vi "StopAllMotion.vi"(0 "System no.":i32, 2 "Has #24":bool=TRUE, 5 "error in (no error)":errorcluster) -> (19 "error out":errorcluster)   [LabVIEW 2020]
doc: "A Support VI to Stop all motion. It takes some controller and syntax specific behavior into account"
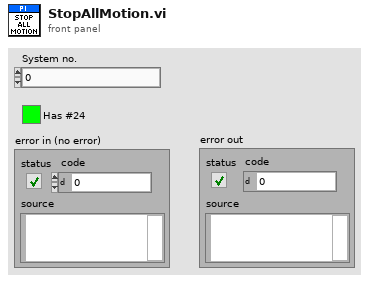
[diagram p1: front panel]
types:
  T1 = typedef "Syntax.ctl" = enum16{"GCS 1.0", "GCS 2.0", "GCS 3.0"}
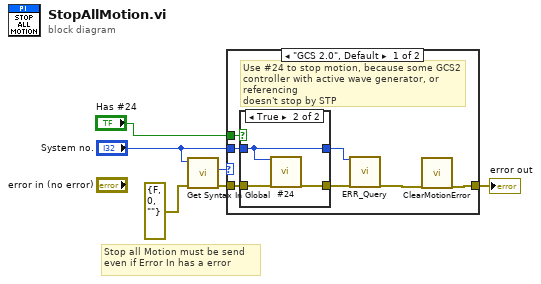
[diagram p0: block diagram]
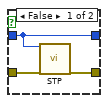
[diagram p2: hidden frame]
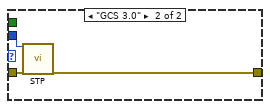
[diagram p3: hidden frame]
diagram:
  # "Stop all Motion must be send\neven if Error In has a error"
  n1 = call "Get Syntax In Global.vi"("error in"=errorcluster {"status"=FALSE, "code"=0, "source"=""}, "System no."="System no.") -> ("error out"=w5:errorcluster, "Syntax"=w4:T1)  [unwired: 8 in]
  n2 = case shown="\"GCS 2.0\", Default" w4 {
    tunnel: [w7 w20] -> w6
    tunnel: "System no." -> [w13 w21]
    tunnel: w5 -> [w12 w22]
    tunnel: "Has #24" -> [w10 _]
    frame "GCS 2.0", Default {
      # "Use #24 to stop motion, because some GCS2 controller with active wave generator, or referencing \ndoesn't stop by STP"
      n3 = case shown="True" w10 {
        tunnel: w13 -> [w14 w17]
        tunnel: w12 -> [w16 w19]
        tunnel: [w15 w18] -> w11
        tunnel: [w14 w17] -> w9
        frame False {
          n4 = call "STP.vi"("System no."=w14, "error in"=w16) -> ("error out"=w15:errorcluster)  [unwired: 17 in]
        }
        frame True {
          n5 = call "#24.vi"("System no."=w17, "error in"=w19) -> ("error out"=w18:errorcluster)  [unwired: 17 out]
        }
      }
      n6 = call "ERR_Query.vi"("System no."=w9, "error in"=w11) -> ("error out"=w8:errorcluster)  [unwired: 17 out]
      n7 = call "ClearMotionError.vi"("error in (no error)"=w8) -> ("error out"=w7:errorcluster)  [unwired: 18 in]
    }
    frame "GCS 3.0" {
      n8 = call "STP.vi"("System no."=w21, "error in"=w22) -> ("error out"=w20:errorcluster)  [unwired: 17 in]
    }
  }
  "error out" <- w6
